vi "MB Serial Slave Demon.vi"(5 "Serial Port Setup (RT Only)":T1(array[cluster]) {"Termination Char" format="%.0x"; "Flow Control" items=["None"=0, "XON/XOFF"=1, "RTS/CTS"=2, "DTR/DSR"=4, "XON/XOFF & RTS/CTS"=3, "XON/XOFF & DTR/DSR"=5]; "Stop Bits" items=["1.0"=10, "1.5"=15, "2.0"=20]; "Data Bits" min=5 max=8 step=1}, 6 "Period":u32=200, 7 "Slave Address":u8 format="%.0x", 9 "Timeouts":u32[](array[numeric]), 10 "Modes":enum16{"RTU", "ASCII"}[](array[ring]), 11 "VISA resource names":string[](array[string])) -> ()   [LabVIEW 2019, in "NI_modbus_upd.lvlib"]
uses:
  NI_modbus_upd.lvlib
  <vilib>/Platform/TimedLoop/XDataNode/timing_clust.ctl
  <vilib>/Platform/TimedLoop/XDataNode/nitl_modes.ctl
  <vilib>/Platform/TimedLoop/XDataNode/wakeup.ctl
  <vilib>/Instr/_visa.llb/VISA Configure Serial Port (Instr).vi
  MB Globals.vi
  <vilib>/platform/TimedLoop/XDataNode/XDataNode.xnode
  <vilib>/Platform/TimedLoop/XDataNode/XDNodeRunTimeDep.lvlib
panel:
  out "Demon Running":bool
  # "VI Name: MB Serial Slave Demon.vi\nPurpose: Modbus Demon"
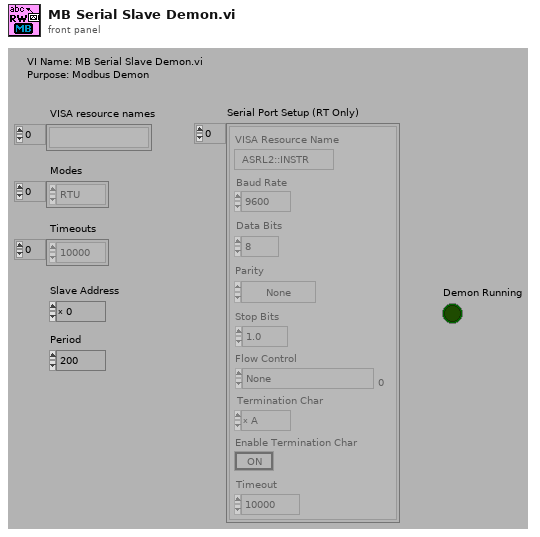
[diagram p1: front panel]
types:
  T1 = cluster{"VISA Resource Name":string, "Baud Rate":u32, "Data Bits":u16, "Parity":enum16{"None", "Odd", "Even", "Mark", "Space"}, "Stop Bits":u16, "Flow Control":u16, "Termination Char":u8, "Enable Termination Char":bool, "Timeout":u32}[]
  T2 = typedef "XDNodeRunTimeDep.lvlib/timing_clust.ctl" = cluster{"Expected End [f-1]":u64, "Actual End [f-1]":u64, "Finished Late? [f-1]":bool, "Expected End [i-1]":u64, "Actual End [i-1]":u64, "Finished Late? [i-1]":bool, "Expected Start [i]":u64, "Actual Start [i]":u64, "Expected Start [f]":u64, "Actual Start [f]":u64, "Source Name":string, "Structure Name":string, "Period":i64, "Deadline":i64, "Offset":i64, "Start":i64, "Priority":i32, "Timeout":i32, "Mode":T3, "Wakeup Reason":T4, "Error":errorcluster, "Source Type":string, "Secondary Source Type":string, "Global End Time":u64, "Global Start Time":u64, "Frame Duration":u64, "Iteration Duration":u64, "Assigned CPU":i32, "I/O Scan Engine Mode":u32}
  T3 = typedef "XDNodeRunTimeDep.lvlib/nitl_modes.ctl" = enum32{"No Change", "Process missed periods, maintain original phase", "Discard missed periods, maintain original phase", "Process missed periods, ignore original phase", "Discard missed periods, ignore original phase"}
  T4 = typedef "XDNodeRunTimeDep.lvlib/wakeup.ctl" = enum32{"Normal", "Aborted", "Asynchronous wakeup", "Timing source error", "Timed loop error", "Timeout"}
  T5 = cluster{"VISA Resource Name":string, "Baud Rate":u32, "Data Bits":u16, "Parity":enum16{"None", "Odd", "Even", "Mark", "Space"}, "Stop Bits":u16, "Flow Control":u16, "Termination Char":u8, "Enable Termination Char":bool, "Timeout":u32}
  T6 = cluster{"Mode":enum16{"RTU", "ASCII"}, "Slave Address":u8}
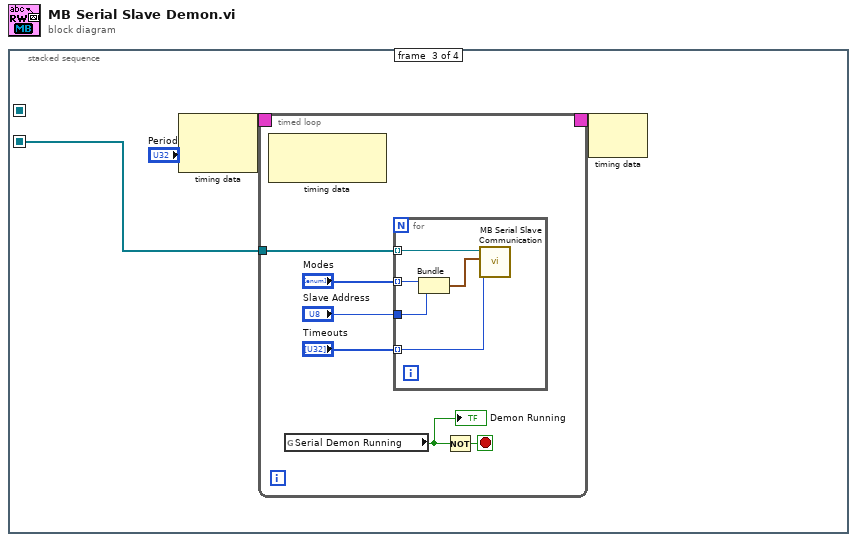
[diagram p0: block diagram]
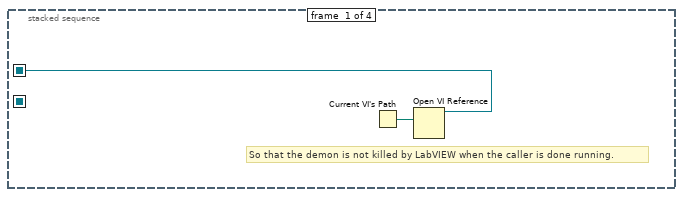
[diagram p2: hidden frame]
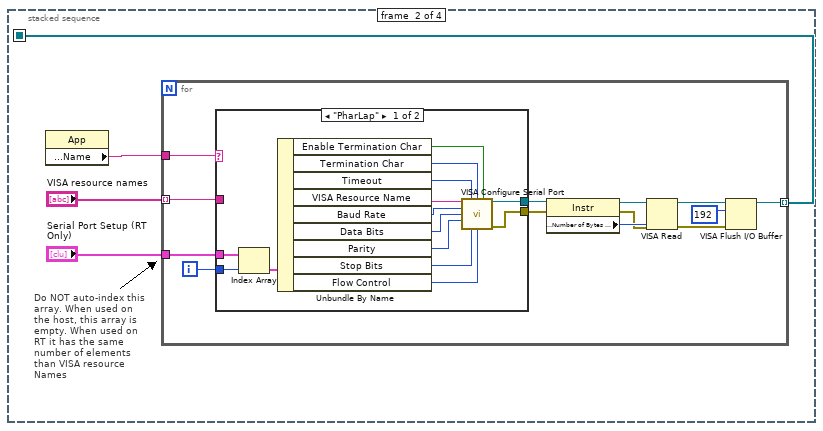
[diagram p3: hidden frame]
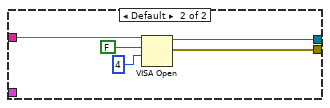
[diagram p4: hidden frame]
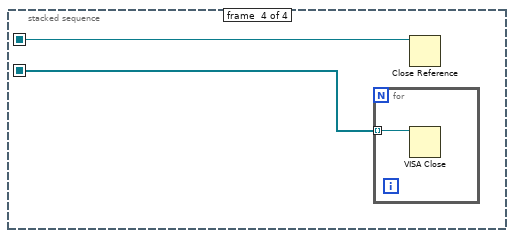
[diagram p5: hidden frame]
diagram:
  n1 = stacked-sequence {
    seq-local: [_ w3 _ _] -> [_ _ w41 w61]
    seq-local: [w1 _ _ _] -> [_ _ _ w60]
    frame #0 {
      # "So that the demon is not killed by LabVIEW when the caller is done running."
      n2 = Current VI's Path() -> (path=w2:path)
      n3 = Open VI Reference(vi path=w2) -> (vi reference=w1:refnum<vi>)  [unwired: 5 in, 1 out]
    }
    frame #1 {
      # "Do NOT auto-index this array. When used on the host, this array is empty. When used on RT it has the same number of elements than VISA resource Names"
      n4 = property class="App"() -> ("Operating System:Name"=w5:string)  [unwired: 2 in, 2 out]
      n5 = for {
        tunnel: "VISA resource names" -> [w11] mode=indexing
        tunnel: [w10] -> w3 mode=indexing
        tunnel: w5 -> [w9]
        tunnel: "Serial Port Setup (RT Only)" -> [w8]
        i -> [w7]
        n6 = case shown="\"PharLap\"" w9 {
          tunnel: [w33 w36] -> w13
          tunnel: [w32 w35] -> w12
          tunnel: w11 -> [_ w34]
          tunnel: w8 -> [w22 _]
          tunnel: w7 -> [w21 _]
          frame "PharLap" {
            n7 = Index Array(array=w22, index=w21) -> (element=w20:T5)
            n8 = Unbundle By Name(w20) -> ("Enable Termination Char"=w26:bool, "Termination Char"=w25:u8, "Timeout"=w27:u32, "VISA Resource Name"=w31:string, "Baud Rate"=w30:u32, "Data Bits"=w29:u16, "Parity"=w28:enum16{"None", "Odd", "Even", "Mark", "Space"}, "Stop Bits"=w24:u16, "Flow Control"=w23:u16)
            n9 = call-poly "VISA Configure Serial Port"("VISA resource name"=w31, "timeout (10sec)"=w27, "termination char\n(0xA = '\\n' = LF)"=w25, "Enable Termination\nChar (T)"=w26, "baud rate (9600)"=w30, "data bits (8)"=w29, "parity (0:none)"=w28, "stop bits (10: 1 bit)"=w24, "flow control (0:none)"=w23) -> ("VISA resource name out"=w33:refnum<visa-resource-name>, "error out"=w32:errorcluster)  [unwired: 5 in]
          }
          frame Default {
            n10 = VISA Open(duplicate session (F)=FALSE, access mode=u32 4, VISA resource name=w34) -> (VISA resource name=w36:refnum<visa-resource-name>, error out=w35:errorcluster)  [unwired: 2 in]
          }
        }
        n11 = property class="Instr"(reference=w13, error in=w12) -> (reference out=w19:refnum<visa-resource-name>, error out=w17:errorcluster, "Serial Settings:Number of Bytes at Serial Port"=w18:u32)
        n12 = VISA Read(VISA resource name=w19, byte count=w18, error in (no error)=w17) -> (VISA resource name out=w14:refnum<visa-resource-name>, error out=w15:errorcluster)  [unwired: 2 out]
        n13 = VISA Flush I/O Buffer(VISA resource name=w14, mask (16)=u16 192, error in (no error)=w15) -> (VISA resource name out=w10:refnum<visa-resource-name>)  [unwired: 1 out]
      }
    }
    frame #2 {
      n14 = node-c288("Period") -> (w39:T2)  [unwired: 1 in]
      n15 = timed-loop {
        tunnel: w41 -> [w45]
        timing-out: [_] -> w40
        timing: w39 -> [_]
        stop <- w44 stop-if-true
        n16 = node-c288() -> ()  [unwired: 1 in, 2 out]
        n17 = global read "MB Globals.vi" "Serial Demon Running"() -> (w43:bool)
        "Demon Running" <- w43
        n18 = for {
          tunnel: "Timeouts" -> [w54] mode=indexing
          tunnel: "Modes" -> [w53] mode=indexing
          tunnel: "Slave Address" -> [w52]
          tunnel: w45 -> [w50] mode=indexing
          n19 = Bundle("Mode"=w53, "Slave Address"=w52) -> (w51:T6)  [unwired: 1 in]
          n20 = call "MB Serial Slave Communication.vi"("Timeout"=w54, "Serial Parameters"=w51, "VISA resource name"=w50) -> ()  [unwired: 7 in, 2 out]
        }
        n21 = Not(x=w43) -> (.not. x?=w44:bool)
      }
      n22 = node-c288(w40) -> ()  [unwired: 1 out]
    }
    frame #3 {
      n23 = for {
        tunnel: w61 -> [w62] mode=indexing
        n24 = VISA Close(VISA resource name=w62) -> ()  [unwired: 1 in, 1 out]
      }
      n25 = Close Reference(reference=w60) -> ()  [unwired: 1 in, 1 out]
    }
  }
